vi "create_log_msg.vi"(10 "string_type":enum16{"none", "csv", "json", "xml"}(ring), 11 "Error in":refnum<class "Error.lvclass">) -> (3 "error_msg_to_log":string)   [LabVIEW 2023, in "Error Handling Interface.lvlib" / "Error.lvclass"]
doc: "Creates a string based on the input Error object (self)\nUse the enum to define the format of the output"
uses:
  Error.lvclass
  Error.lvclass/Error.ctl
  error_type.ctl
  29e50747-ab6d-4b85-8b93-7d186a773c3d.vi
  <vilib>/JDP Science/JSONtext/Variant to JSON Text.vi
  <vilib>/JDP Science/JSONtext/LVClass Serializer/JSONtext LVClass Serializer.lvclass
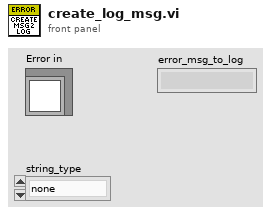
[diagram p1: front panel]
types:
  T1 = typedef "Error Handling Interface.lvlib/Error.lvclass/error_type.ctl" = enum16{"FATAL", "ERROR", "WARNING", "INFO", "DEBUG", "TRACE"}
  T2 = cluster{"error_time":timestamp, "error_type":T1, "error_source_object":string, "error_mark":string, "code":i32, "source":string}
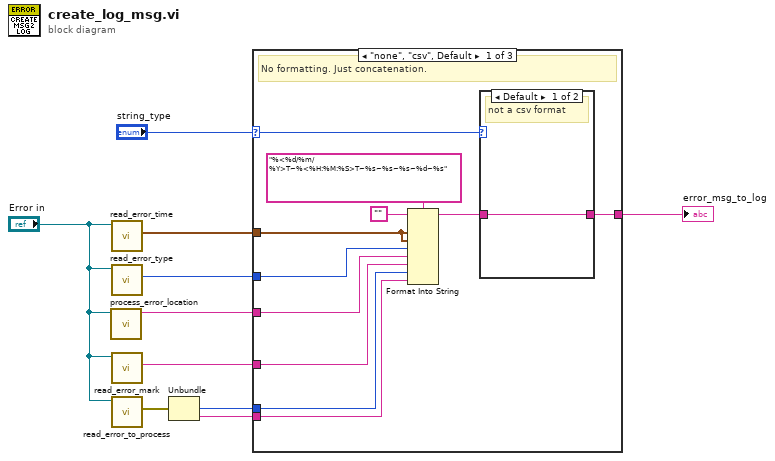
[diagram p0: block diagram]
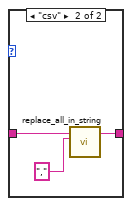
[diagram p2: hidden frame]
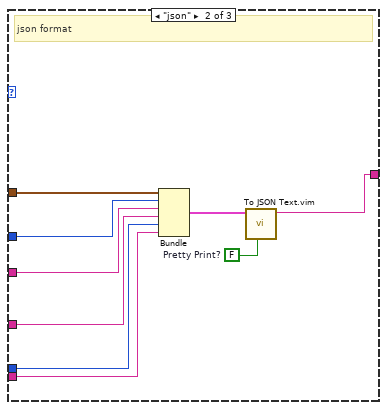
[diagram p3: hidden frame]
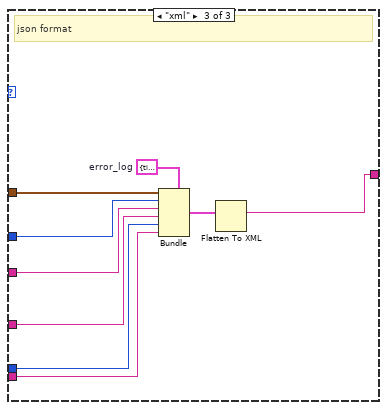
[diagram p4: hidden frame]
diagram:
  n1 = call "process_error_location.vi"("Error in"="Error in") -> ("error_source_object"=w8:string)  [unwired: 10 in]
  n2 = call "read_error_time.vi"("Error in"="Error in") -> ("error_time"=w5:timestamp)  [unwired: 10 in]
  n3 = call "read_error_type.vi"("Error in"="Error in") -> ("error_type"=w4:T1)  [unwired: 10 in]
  n4 = call "read_error_mark.vi"("Error in"="Error in") -> ("error_mark"=w6:string)  [unwired: 10 in]
  n5 = call "read_error_to_process.vi"("Error in"="Error in") -> ("error_to_process"=w3:errorcluster)  [unwired: 10 in]
  n6 = Unbundle(w3) -> ("code"=w2:i32, "source"=w1:string)  [unwired: 1 out]
  n7 = case shown="\"none\", \"csv\", Default" "string_type" {
    selector: "string_type" -> [w13 _ _]
    tunnel: w8 -> [w21 w32 w41]
    tunnel: [w14 w27 w36] -> w7
    tunnel: w6 -> [w20 w31 w40]
    tunnel: w5 -> [w11 w34 w43]
    tunnel: w4 -> [w12 w33 w42]
    tunnel: w2 -> [w19 w30 w39]
    tunnel: w1 -> [w18 w29 w38]
    frame "none", "csv", Default {
      # "No formatting. Just concatenation."
      n8 = Format Into String(format string="%<%d/%m/%Y>T~%<%H:%M:%S>T~%s~%s~%s~%d~%s", initial string="", w11, w11, w12, w21, w20, w19, w18) -> (resulting string=w15:string)  [unwired: 1 in, 1 out]
      n9 = case shown="Default" w13 {
        tunnel: w15 -> [w22 w25]
        tunnel: [w22 w24] -> w14
        frame Default {
          # "not a csv format"
        }
        frame "csv" {
          n10 = call "replace_all_in_string.vi"("replace_string"="," ("replace string (\"\")"), "string_in"=w25) -> ("string_out"=w24:string)  [unwired: 9 in]
        }
      }
    }
    frame "json" {
      w26 = FALSE  # Pretty Print?
      # "json format"
      n11 = Bundle("error_time"=w34, "error_type"=w33, "error_source_object"=w32, "error_mark"=w31, "code"=w30, "source"=w29) -> (w28:T2)  [unwired: 1 in]
      n12 = call "To JSON Text.vim"("Pretty Print?"=w26, "Anything"=w28) -> ("<JSON>"=w27:string)  [unwired: 8 in, 1 out]
    }
    frame "xml" {
      w35 = T2 {"error_time"=timestamp(0 s since 1904-01-01), "error_type"=enum."FATAL", "error_source_object"="", "error_mark"="", "code"=0, "source"=""}  # error_log
      # "json format"
      n13 = Bundle(cluster=w35, "error_time"=w43, "error_type"=w42, "error_source_object"=w41, "error_mark"=w40, "code"=w39, "source"=w38) -> (w37:T2)
      n14 = Flatten To XML(6:w37) -> (2:w36:string)
    }
  }
  "error_msg_to_log" <- w7
